vi "AB_Engine_Build.vi"(6 "progressBarEvents":T3, 7 "Programmatic":bool, 8 "error in (no error)":errorcluster, 9 "Build operation":T5, 10 "ContextForBuild in":refnum<vi>, 11 "Object":T6) -> (0 "error out":errorcluster, 2 "Dependencies":T1[](array[typedef]), 3 "GeneratedFiles out":path[](array[path]), 4 "GeneratedFileGUIDs":string[](array[string]), 5 "OutputDirectory":path)   [LabVIEW 2020]
uses:
  <resource>/Framework/Providers/API/ItemRef.ctl
  <vilib>/AppBuilder/Engine/AB_Engine_Operation.ctl
  <resource>/Framework/Providers/Common/provcom_ProgressBar_Events.ctl
  <resource>/Framework/Providers/API/mxLvBuildError.ctl
  <vilib>/AppBuilder/AB_Dependency.ctl
  <vilib>/Utility/lvfile.llb/LVFileType.ctl
  <vilib>/AppBuilder/AB_Classes/Build/AB_Build.lvclass
  <vilib>/Utility/lvfile.llb/NI_FileType.lvlib
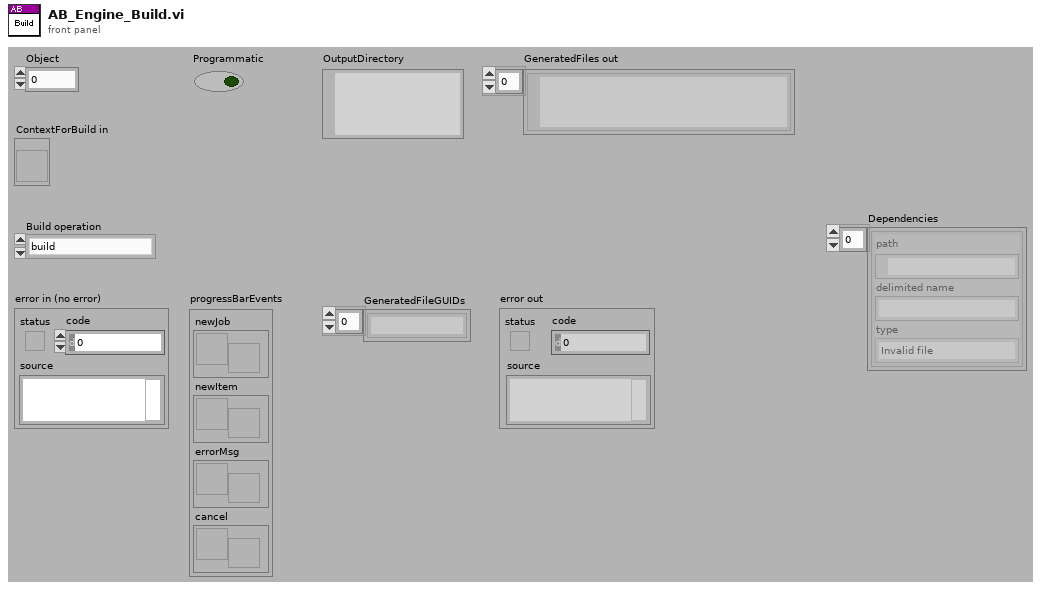
[diagram p1: front panel]
types:
  T1 = typedef "AB_Dependency.ctl" = cluster{"path":path, "delimited name":string, "type":T2}
  T2 = typedef "NI_FileType.lvlib/LVFileType.ctl" = enum32{"Invalid file", "Unknown type", "Instrument", "Control", "Polymorphic VI", "Project", "Library", "LVClass", "XControl", "XNode", "Shared library", ".NET assembly", "ActiveX interface", "CIN", "Run-time menu", "Palette menu", "Help file", "LLB", "XNode Edit Dependency", "Class Private Data Control", "Statechart", "MathScript .m file", "Ladder Diagram", "LVLibp", "XNode Build Dependency"}
  T3 = typedef "provcom_ProgressBar_Events.ctl" = cluster{"newJob":refnum<user-event>, "newItem":refnum<user-event>, "errorMsg":T4, "cancel":refnum<user-event>}
  T4 = typedef "mxLvBuildError.ctl" = refnum<user-event>
  T5 = typedef "AB_Engine_Operation.ctl" = enum16{"build", "preview", "installer preview"}
  T6 = typedef "ItemRef.ctl" = u64
  T7 = typedef "AB_Build.ctl" = cluster{"buildSpecName":string, "buildSpecDescription":string, "destinations":refnum<class "AB_Destination.lvclass">[], "exclusionOption":T8, "defaultLanguage":string, "supportedLanguages":string[], "excludedDirectories":path[], "buildContext":refnum<vi>, "buildObject":T6, "preview":bool, "programatic":bool, "progressBarEvents":T3, "userLog_Path":path, "preActionID":string, "preAction_Path":path, "postActionID":string, "postAction_Path":path, "eng_checkForBrokenVIs?":bool, "eng_verboseLinkerErrors?":bool, "localDest_Path":path, "targetDest_Path":path, "removeVIObject":u16, "cache":refnum<class "PreviewCache.lvclass">, "use cache":bool, "previewCache_ID":string, "buildCache_ID":string, "eng_TempLocalDest_Path":path, "eng_collectDependencies?":bool, "versionInfo":cluster{"buildVersion":cluster{"major":u16, "minor":u16, "patch":u16, "build":u16}, "autoIncrement":bool}, "eng_enableVIChecksums":bool}
  T8 = typedef "AB_Exclusion_Option.ctl" = cluster{"typedefs":bool, "polymorphicVIs":bool, "unusedLibraryItems":bool, "modifyLibraryFile":bool, "edit-timeDependencies":bool, "inlineVIs":bool, "dependent PPLs":bool, "dependent DLLs":bool}
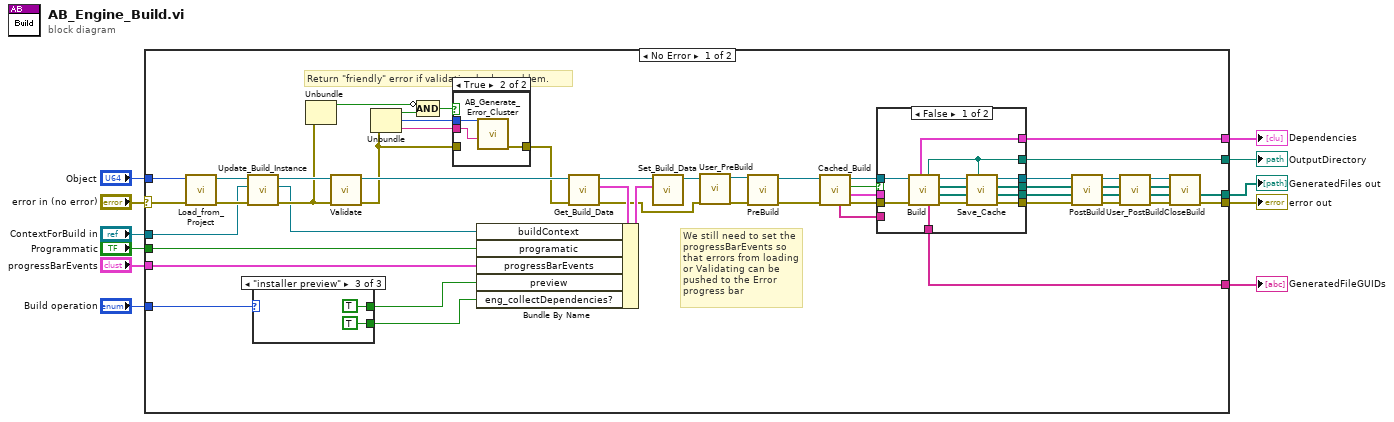
[diagram p0: block diagram]
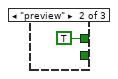
[diagram p3: hidden frame]
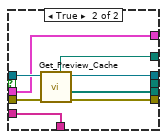
[diagram p4: hidden frame]
diagram:
  n1 = case shown="No Error" "error in (no error)" {
    selector: "error in (no error)" -> [w50 w92]
    tunnel: [w59 _] -> w11
    tunnel: [w58 w92] -> w2
    tunnel: "Object" -> [w57 _]
    tunnel: "ContextForBuild in" -> [w36 _]
    tunnel: "Build operation" -> [w14 _]
    tunnel: "Programmatic" -> [w52 _]
    tunnel: "progressBarEvents" -> [w51 _]
    tunnel: [w49 _] -> w4
    tunnel: [w48 _] -> w3
    tunnel: [w17 _] -> w1
    frame No Error {
      # "Return \"friendly\" error if validation had a problem."
      # "We still need to set the progressBarEvents so that errors from loading or Validating can be  pushed to the Error progress bar"
      n2 = call <vilib>:"Load_from_Project.vi"("error in (no error)"=w50, "Object"=w57) -> ("error out"=w38:errorcluster, "Build out"=w40:refnum<class "AB_Build.lvclass">)  [unwired: 8 out]
      n3 = call-dynamic "Update_Build_Instance.vi"("error in (no error)"=w38, "AppInstanceForBuild in"=w36, "Build in"=w40) -> ("error out"=w37:errorcluster, "AppInstanceForBuild out"=w35:refnum<vi>, "Build out"=w39:refnum<class "AB_Build.lvclass">)  [unwired: 6 out]
      n4 = case shown="\"installer preview\"" w14 {
        tunnel: [_ TRUE TRUE] -> w13
        tunnel: [_ _ TRUE] -> w12
        frame "build", Default {
        }
        frame "preview" {
        }
        frame "installer preview" {
        }
      }
      n5 = Unbundle(w37) -> ("status"=w46:bool)  [unwired: 2 out]
      n6 = call-dynamic "Validate.vi"("error in (no error)"=w37, "Build in"=w39) -> ("error out"=w42:errorcluster, "Build out"=w53:refnum<class "AB_Build.lvclass">)  [unwired: 8 out]
      n7 = Unbundle(w42) -> ("status"=w47:bool, "code"=w44:i32, "source"=w43:string)
      n8 = Compound Arithmetic op=AND(invert w46, w47) -> (w45:bool)
      n9 = case shown="True" w45 {
        tunnel: w44 -> [_ w91]
        tunnel: w43 -> [_ w90]
        tunnel: w42 -> [w88 _]
        tunnel: [w88 w89] -> w41
        frame False {
        }
        frame True {
          n10 = call <vilib>:"AB_Generate_Error_Cluster.vi"("Additional Message"=w90, "Code"=w91) -> ("error out"=w89:errorcluster)  [unwired: 2 in, 7 out]
        }
      }
      n11 = call <vilib>:"Get_Build_Data.vi"("error in (no error)"=w41, "Class in"=w53) -> ("error out"=w26:errorcluster, "data"=w56:T7, "Class out"=w54:refnum<class "AB_Build.lvclass">)  [unwired: 7 out]
      n12 = Bundle By Name(cluster=w56, "buildContext"=w35, "programatic"=w52, "progressBarEvents"=w51, "preview"=w13, "eng_collectDependencies?"=w12) -> (w55:T7)
      n13 = call <vilib>:"Set_Build_Data.vi"("data"=w55, "Class in"=w54) -> ("Class out"=w25:refnum<class "AB_Build.lvclass">)  [unwired: 1 in, 8 out]
      n14 = call-dynamic "User_PreBuild.vi"("error in (no error)"=w26, "Build in"=w25) -> ("error out"=w23:errorcluster, "Build out"=w24:refnum<class "AB_Build.lvclass">)  [unwired: 8 in]
      n15 = call-dynamic "PreBuild.vi"("error in (no error)"=w23, "Build in"=w24) -> ("error out"=w21:errorcluster, "Build out"=w22:refnum<class "AB_Build.lvclass">)  [unwired: 1 in, 7 out]
      n16 = call-dynamic "Cached_Build.vi"("error in (no error)"=w21, "AB_Build in"=w22) -> ("error out"=w18:errorcluster, "Dependencies"=w16:T1[], "valid?"=w19:bool, "AB_Build out"=w20:refnum<class "AB_Build.lvclass">, "GeneratedFileGUIDs"=w15:string[])  [unwired: 5 in]
      n17 = case shown="False" w19 {
        tunnel: w20 -> [w79 w86]
        tunnel: w18 -> [w78 w85]
        tunnel: [w76 w87] -> w63
        tunnel: [w75 w84] -> w62
        tunnel: [w71 _] -> w61
        tunnel: [w72 w82] -> w60
        tunnel: [w67 w80] -> w49
        tunnel: [w69 w83] -> w48
        tunnel: [w68 w81] -> w17
        tunnel: w16 -> [_ w81]
        tunnel: w15 -> [_ w80]
        frame False {
          n18 = call-dynamic "Build.vi"("error in (no error)"=w78, "Build in"=w79) -> ("error out"=w74:errorcluster, "GeneratedFiles"=w73:path[], "GeneratedDirectories"=w70:path[], "Build out"=w77:refnum<class "AB_Build.lvclass">, "GeneratedFileGUIDs"=w67:string[], "OutputDirectory"=w69:path, "Dependencies"=w68:T1[])  [unwired: 1 in, 2 out]
          n19 = call <vilib>:"Save_Cache.vi"("OutputDirectory"=w69, "error in (no error)"=w74, "GeneratedFiles"=w73, "GeneratedDirectories"=w70, "AB_Build in"=w77) -> ("error out"=w75:errorcluster, "GeneratedFiles out"=w72:path[], "GeneratedDirectories out"=w71:path[], "AB_Build out"=w76:refnum<class "AB_Build.lvclass">)  [unwired: 3 in]
        }
        frame True {
          n20 = call <vilib>:"Get_Preview_Cache.vi"("error in (no error)"=w85, "AB_Build in"=w86) -> ("error out"=w84:errorcluster, "GeneratedFiles"=w82:path[], "AB_Build out"=w87:refnum<class "AB_Build.lvclass">, "OutputDirectory"=w83:path)  [unwired: 6 in]
        }
      }
      n21 = call-dynamic "PostBuild.vi"("error in (no error)"=w62, "GeneratedFiles in"=w60, "GeneratedDirectories in"=w61, "Build in"=w63) -> ("error out"=w34:errorcluster, "GeneratedFiles out"=w27:path[], "GeneratedDirectories out"=w30:path[], "Build out"=w31:refnum<class "AB_Build.lvclass">)  [unwired: 4 out]
      n22 = call-dynamic "User_PostBuild.vi"("error in (no error)"=w34, "GeneratedFiles in"=w27, "GeneratedDirectories in"=w30, "Build in"=w31) -> ("error out"=w33:errorcluster, "GeneratedFiles out"=w28:path[], "GeneratedDirectories out"=w29:path[], "Build out"=w32:refnum<class "AB_Build.lvclass">)  [unwired: 4 in]
      n23 = call-dynamic "CloseBuild.vi"("error in (no error)"=w33, "GeneratedFiles"=w28, "GeneratedDirectories"=w29, "Build in"=w32) -> ("error out"=w58:errorcluster, "GeneratedFiles out"=w59:path[])  [unwired: 6 out]
    }
    frame Error {
    }
  }
  "error out" <- w2
  "GeneratedFiles out" <- w11
  "GeneratedFileGUIDs" <- w4
  "OutputDirectory" <- w3
  "Dependencies" <- w1
